vi "Redraw Window.vi"(8 "error in":errorcluster caption="error in (no error)" {"code" format="%d\n%x"}, 11 "window refnum":T1) -> (0 "error out":errorcluster {"code" format="%d\n%x"}, 3 "window refnum out":T1)   [LabVIEW 2020, in "MacroAssert.lvlib" / "Win Util New.lvlib"]
uses:
  Win Util New.lvlib
  Window Refnum.ctl
  user32.dll
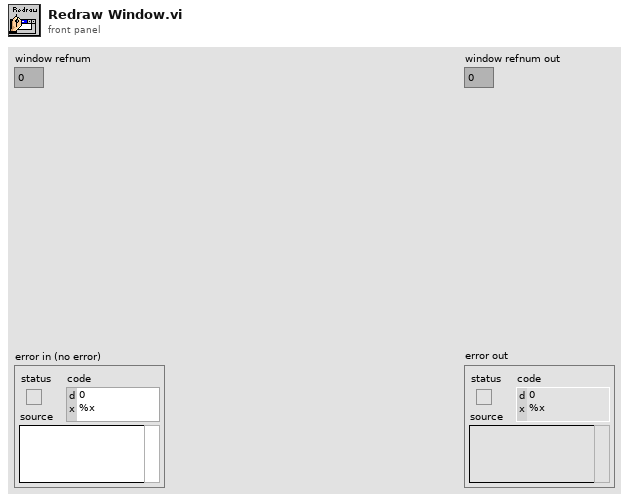
[diagram p1: front panel]
types:
  T1 = typedef "MacroAssert.lvlib/Win Util New.lvlib/Window Refnum.ctl" = u64
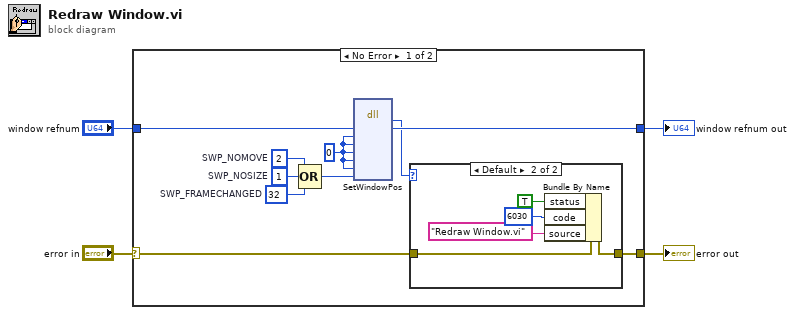
[diagram p0: block diagram]
diagram:
  n1 = case shown="No Error" "error in" {
    selector: "error in" -> [w12 w22]
    tunnel: [w13 w22] -> w4
    tunnel: [w10 w21] -> w3
    tunnel: "window refnum" -> [w11 w21]
    frame No Error {
      w7 = u32 2  # SWP_NOMOVE
      w8 = u32 1  # SWP_NOSIZE
      w6 = u32 32  # SWP_FRAMECHANGED
      w5 = 0
      n2 = Compound Arithmetic op=OR(w7, w8, w6) -> (w14:u32)
      n3 = dll-call lib="USER32.DLL" fn="SetWindowPos"("hWnd"=w11, "hWndInsertAfter"=w5, "left"=w5, "top"=w5, "width"=w5, "height"=w5, "fuFlags"=w14) -> ("error"=w9:i32, "hWnd"=w10:u64)  [unwired: 8 in, 3 out]
      n4 = case shown="Default" w9 {
        tunnel: [w15 w19] -> w13
        tunnel: w12 -> [w15 w18]
        frame 0 {
        }
        frame Default {
          n5 = Bundle By Name(cluster=w18, "status"=TRUE, "code"=6030, "source"="Redraw Window.vi") -> (w19:errorcluster)
        }
      }
    }
    frame Error {
    }
  }
  "window refnum out" <- w3
  "error out" <- w4
